vi "Get INI Refnum.vi"() -> (3 "INI Refnum Out":T1)   [LabVIEW 2014, in "Standard Editor.lvlib" / "DCAF INI.lvlib"]
doc: "Get INI Refnum from fgv_DCAF INI Refnum.vi"
uses:
  DCAF INI.lvlib
  <vilib>/Utility/config.llb/Config Data RefNum.ctl
  enum_DCAF INI FGV Action.ctl
  <vilib>/Utility/config.llb/NI_LVConfig.lvlib
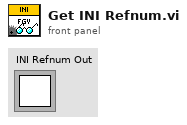
[diagram p1: front panel]
types:
  T1 = typedef "NI_LVConfig.lvlib/Config Data RefNum.ctl" = refnum<k1>
  T2 = typedef "Standard Editor.lvlib/DCAF INI.lvlib/enum_DCAF INI FGV Action.ctl" = enum16{"Get", "Set"}
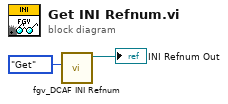
[diagram p0: block diagram]
diagram:
  n1 = call "fgv_DCAF INI Refnum.vi"("Action"=enum_DCAF_INI_FGV_Action."Get") -> ("INI Refnum Out"=→"INI Refnum Out":T1)  [unwired: 10 in]
